vi "queu-variable-size-array.vi"() -> ()   [LabVIEW 2015]
panel:
  out "Array 3":dbl[](array[numeric])
  out "initialized array":dbl[](array[numeric])
  out "element 2":dbl[](array[numeric])
  out "Array 2":dbl[][](array[numeric])
  out "Array":dbl[][](array[numeric])
  # "THe question this vi seeks to answer is:\nHow does the queu producer-consumer handle variable size arrays?"
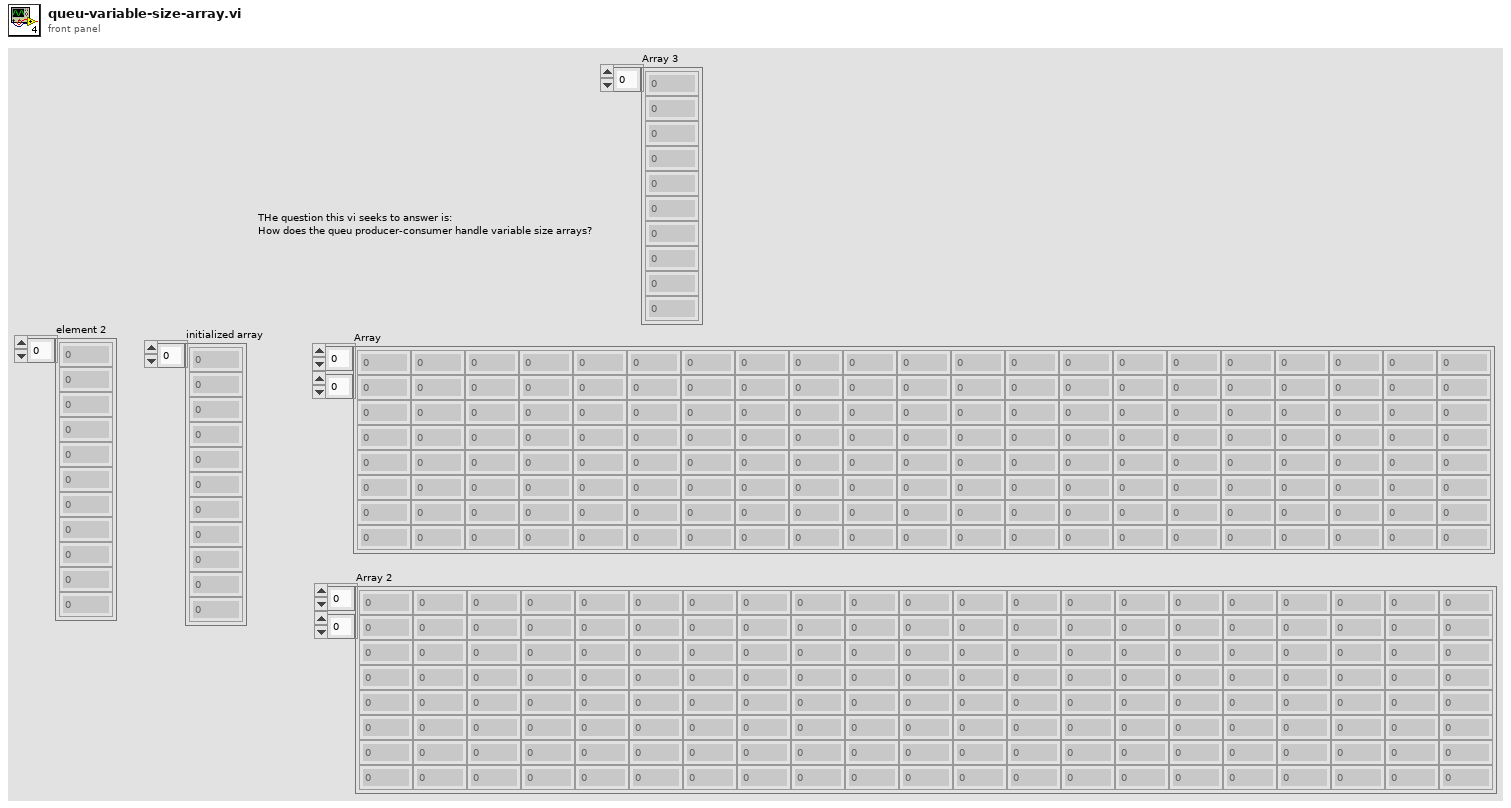
[diagram p1: front panel]
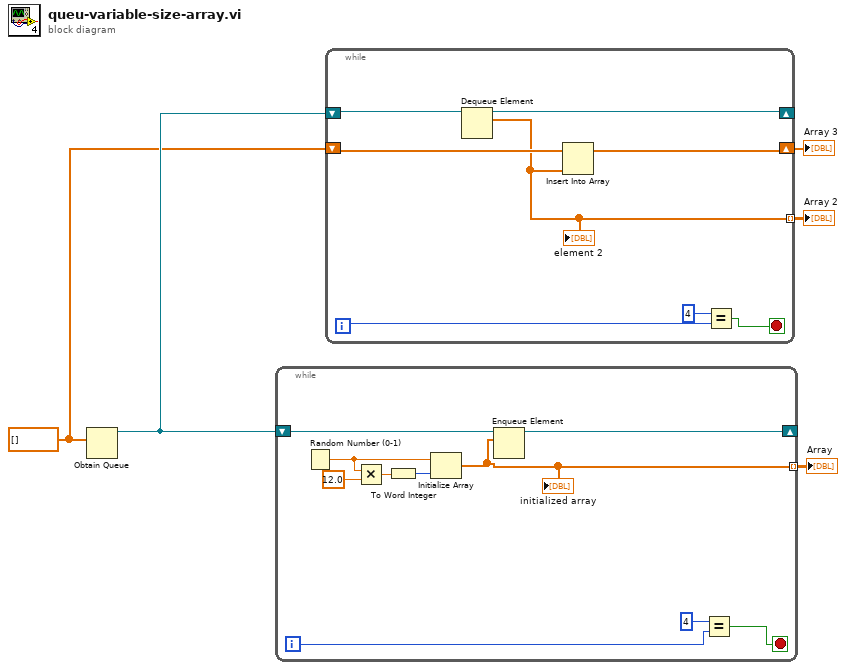
[diagram p0: block diagram]
diagram:
  w2 = dbl[] []
  n1 = Obtain Queue(element data type=w2) -> (queue out=w5:refnum<queue>)  [unwired: 4 in, 2 out]
  n2 = while {
    shift-right: [w14] -> _
    shift-left: w5 -> [w15]
    tunnel: [w9] -> w4 mode=indexing
    i -> [w6]
    stop <- w7 stop-if-true
    n3 = Random Number (0-1)() -> (number: 0 to 1=w11:dbl)
    n4 = Multiply(x=w11, y=12.0) -> (x*y=w12:dbl)
    n5 = To Word Integer(number=w12) -> (16bit integer=w13:i16)
    n6 = Initialize Array(w11, w13) -> (w9:dbl[])
    "initialized array" <- w9
    n7 = Enqueue Element(queue=w15, element=w9) -> (queue out=w14:refnum<queue>)  [unwired: 2 in, 2 out]
    n8 = Equal?(x=4, y=w6) -> (x = y?=w7:bool)
  }
  "Array" <- w4
  n9 = while {
    shift-right: [w22] -> _
    shift-left: w5 -> [w23]
    tunnel: [w16] -> w3 mode=indexing
    shift-right: [w17] -> w1
    shift-left: w2 -> [w18]
    i -> [w20]
    stop <- w21 stop-if-true
    n10 = Dequeue Element(queue=w23) -> (queue out=w22:refnum<queue>, element=w16:dbl[])  [unwired: 2 in, 2 out]
    "element 2" <- w16
    n11 = Insert Into Array(array=w18, new element=w16) -> (w17:dbl[])  [unwired: 1 in]
    n12 = Equal?(x=4, y=w20) -> (x = y?=w21:bool)
  }
  "Array 2" <- w3
  "Array 3" <- w1
